vi "1100945.vi"() -> ()   [LabVIEW 2019]
uses:
  <vilib>/vision/driver/NI_Vision_Acquisition_Software.lvlib
  <vilib>/userDefined/High Color/IMAQdx.ctl
panel:
  out "Main color 2":string
  out "RGB Array 2":dbl[](array[numeric])
  in  "stop":bool
  out "Image":T1(plugin-control)
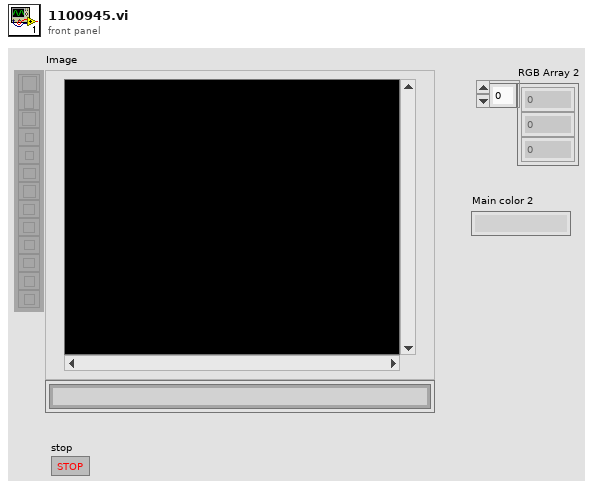
[diagram p1: front panel]
types:
  T1 = typedef "IMAQ Image.ctl" = refnum<image>
  T2 = typedef "IMAQdx.ctl" = refnum<k21>
  T3 = typedef "eventvkey.ctl" = enum16{"ASCII", "Enter", "Return", "Shift", "Ctrl", "Alt", "Cmd", "Opt", "Caps", "NumLock", "Clear", "Break", "Up", "Down", "Left", "Right", "Insert", "Delete", "Home", "End", "PageUp", "PageDown", "Escape", "Help", "Pause", "ScrollLock", "F1", "F2", "F3", "F4", "F5", "F6", "F7", "F8", "F9", "F10", "F11", "F12", "F13", "F14", "F15", "F16", "F17", "F18", "F19", "F20", "F21", "F22", "F23", "F24", "Play", "VolumeUp", "VolumeDown", "Mute", "Two Byte Char"}
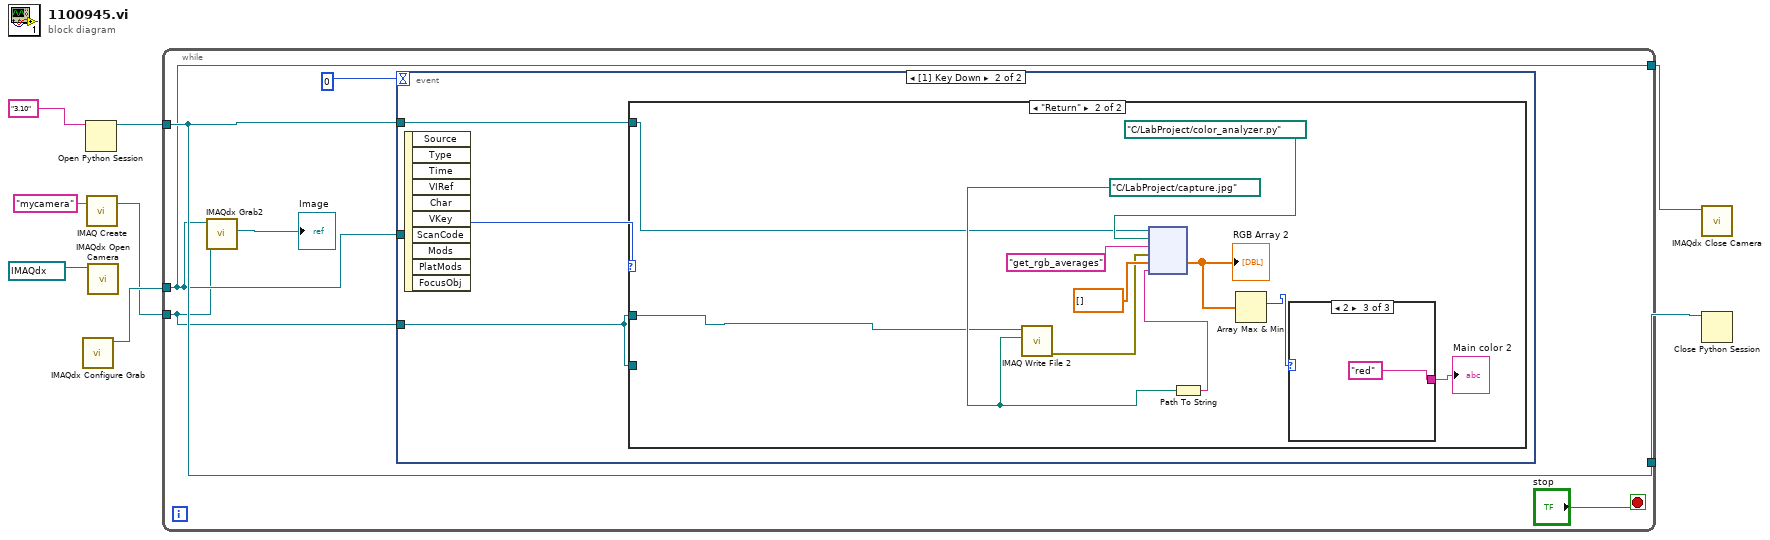
[diagram p0: block diagram]
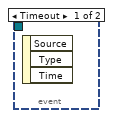
[diagram p2: hidden frame]
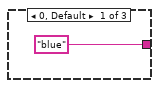
[diagram p4: hidden frame]
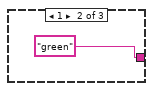
[diagram p5: hidden frame]
diagram:
  n1 = call <vilib>:"IMAQdx Configure Grab.vi"() -> ("Session Out"=w8:T2)  [unwired: 10 in, 1 out]
  n2 = Open Python Session(python version="3.10" ("Python version")) -> (session out=w4:refnum<k35>)  [unwired: 2 in, 1 out]
  n3 = call "IMAQ Create"("Image Name"="mycamera") -> ("New Image"=w6:T1)  [unwired: 4 in, 1 out]
  n4 = call <vilib>:"IMAQdx Open Camera.vi"("Session In"=T2 "cam0") -> ()  [unwired: 9 in, 2 out]
  n5 = while {
    tunnel: w8 -> [w11]
    tunnel: w6 -> [w10]
    tunnel: w4 -> [w13]
    tunnel: [w11] -> w3
    tunnel: [w13] -> w2
    stop <- "stop" stop-if-true
    n6 = call <vilib>:"IMAQdx Grab2.vi"("Image In"=w10, "Session In"=w11) -> ("Image Out"=→"Image":T1)  [unwired: 6 in, 3 out]
    n7 = event shown="[1] Key Down" {
      selector: _ -> [_ _]
      dyn-events: _ -> [_ _]
      timeout: u32 0 ("Time") -> [_ _]
      tunnel: w13 -> [_ w16]
      tunnel: w11 -> [_ _]
      tunnel: w10 -> [_ w15]
      event Timeout {
        n8 = event-data() -> ()  [unwired: 1 in, 3 out]
      }
      event Key Down {
        n9 = event-data() -> ("VKey"=w17:T3)  [unwired: 1 in, 9 out]
        n10 = case shown="\"Return\"" w17 {
          tunnel: w16 -> [_ w20]
          tunnel: w15 -> [_ _]
          tunnel: w15 -> [_ w19]
          frame "ASCII", Default {
          }
          frame "Return" {
            w21 = path "C:/LabProject/capture.jpg" ("File Path")
            n11 = call-poly "IMAQ Write File 2"("File Path"=w21, "Image"=w19) -> ("error out"=w23:errorcluster)  [unwired: 8 in, 1 out]
            n12 = Path To String(path=w21) -> (string=w26:string)
            n13 = node(w20, path "C:/LabProject/color_analyzer.py" ("module path"), "get_rgb_averages" ("function name"), w23, dbl[] [], w26) -> (w25:dbl[])  [unwired: 1 in, 4 out]
            "RGB Array 2" <- w25
            n14 = Array Max & Min(array=w25) -> (max index (indices)=w18:i32)  [unwired: 3 out]
            n15 = case shown="2" w18 {
              tunnel: ["blue" "green" "red"] -> w24
              frame 0, Default {
              }
              frame 1 {
              }
              frame 2 {
              }
            }
            "Main color 2" <- w24
          }
        }
      }
    }
  }
  n16 = call <vilib>:"IMAQdx Close Camera.vi"("Session In"=w3) -> ()  [unwired: 10 in, 1 out]
  n17 = Close Python Session(session in=w2) -> ()  [unwired: 1 in, 1 out]
